vi "_6Unv_Gates.vi"() -> ()   [LabVIEW 2018]
panel:
  out "LED2":bool
  out "LED1":bool
  in  "i2":bool
  in  "i1":bool
  in  "i2":bool
  in  "i1":bool
  # "NAND Logic"
  # "NOR Logic"
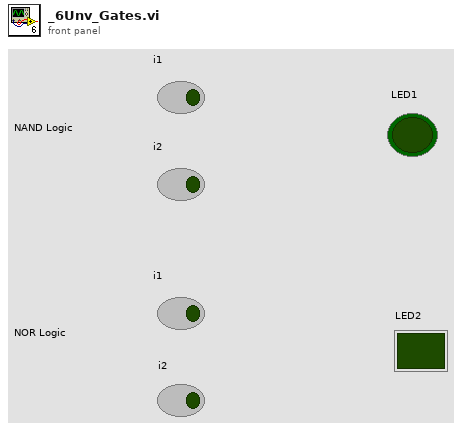
[diagram p1: front panel]
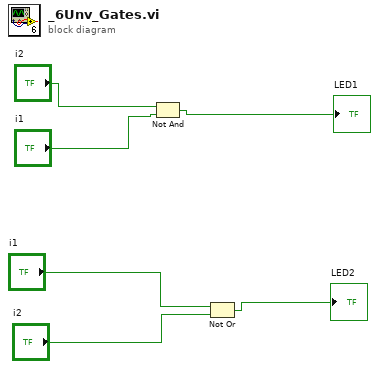
[diagram p0: block diagram]
diagram:
  n1 = Not And(1:"i1", 2:"i2") -> (0:→"LED1":bool)
  n2 = Not Or(1:"i2", 2:"i1") -> (0:→"LED2":bool)
